vi "Wafer_Map_Suss_Prober_Index.vi"(8 "error in (no error)":errorcluster, 11 "RegistrationNumber":T1) -> (0 "error out":errorcluster, 1 "ResponseString 2":string, 3 "RegistrationNumber out":T1, 4 "End Of Wafer":bool)   [LabVIEW 2012]
uses:
  <instrlib>/SUSSProberInterface/SussProberInterface.llb/RegistrationNumber.ctl
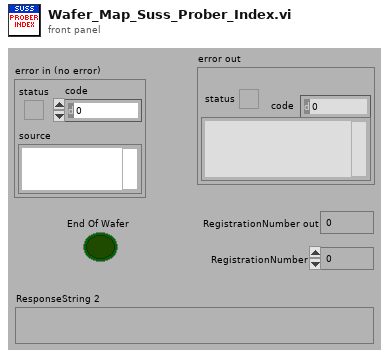
[diagram p1: front panel]
types:
  T1 = typedef "RegistrationNumber.ctl" = i32
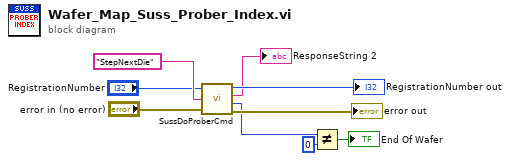
[diagram p0: block diagram]
diagram:
  n1 = call <instrlib>:"SussDoProberCmd.vi"("RegistrationNumber in"="RegistrationNumber", "CommandString"="StepNextDie" ("Actuator 2"), "error in"="error in (no error)") -> ("RegistrationNumber out"=→"RegistrationNumber out":T1, "ResponseString"=→"ResponseString 2":string, "ProberBenchErrorCode"=w8:i32, "error out"=→"error out":errorcluster)
  n2 = Not Equal?(x=w8, y=0) -> (x != y?=→"End Of Wafer":bool)
